vi "Bundle Script_In Place Insert.vi"(6 "Action Choice In":enum32{"Choice 1", "Choice 2"}(radio), 8 "error in":errorcluster, 10 "Selected Items Tags":string[](array[string]), 11 "Affected Items":T1) -> (0 "error out":errorcluster)   [LabVIEW 2023]
uses:
  top/BundleMagic.ctl
panel:
  # "Choice 1 is before, Choice 2 is after"
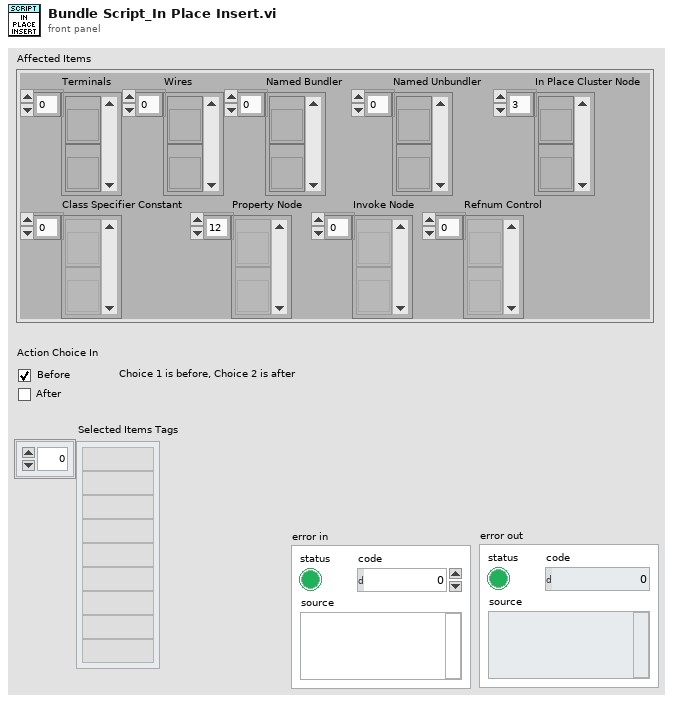
[diagram p1: front panel]
types:
  T1 = typedef "BundleMagic.ctl" = cluster{"Terminals":refnum<vi>[], "Wires":refnum<vi>[], "Named Bundler":refnum<vi>[], "Named Unbundler":refnum<vi>[], "In Place Cluster Node":refnum<vi>[], "Class Specifier Constant":refnum<vi>[], "Property Node":refnum<vi>[], "Invoke Node":refnum<vi>[], "Refnum Control":refnum<vi>[]}
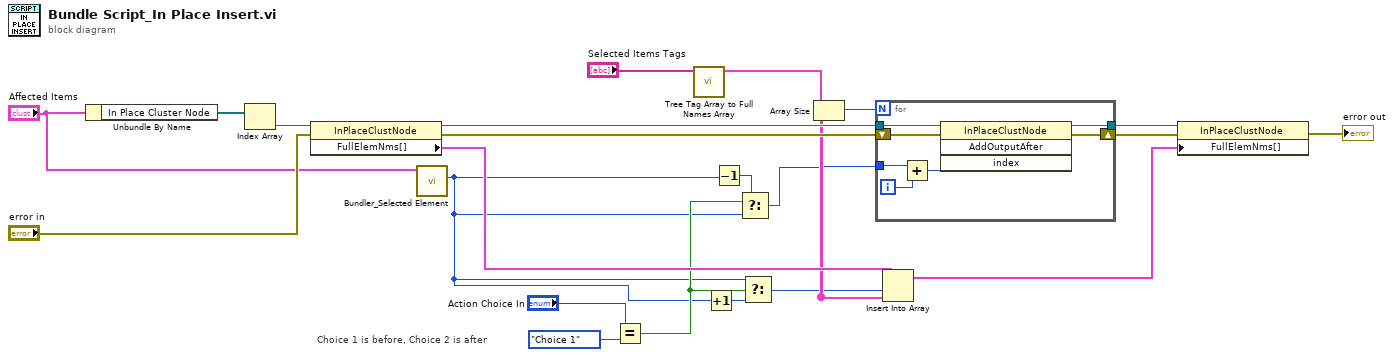
[diagram p0: block diagram]
diagram:
  # "Choice 1 is before, Choice 2 is after"
  n1 = Unbundle By Name("Affected Items") -> ("In Place Cluster Node"=w22:refnum<vi>[])
  n2 = Index Array(array=w22) -> (element=w19:refnum<vi>)  [unwired: 1 in]
  n3 = property class="InPlaceClustNode"(reference=w19, error in="error in") -> (reference out=w20:refnum<vi>, error out=w16:errorcluster, "FullElemNms[]"=w17:cluster{string[]}[])
  n4 = call "Bundler_Selected Element.vi"("Affected Items"="Affected Items") -> ("index of element"=w1:i32)  [unwired: 5 in, 5 out]
  n5 = Equal?(x="Action Choice In", y=enum32{"Choice 1", "Choice 2"}."Choice 1" ("Action Choice In")) -> (x = y?=w3:bool)
  n6 = call "Tree Tag Array to Full Names Array.vi"("Selected Items Tags"="Selected Items Tags") -> ("Tree Item Values (nested form)"=w13:cluster{"Array":string[]}[])  [unwired: 6 in, 4 out]
  n7 = Increment(x=w1) -> (x+1=w4:i32)
  n8 = Decrement(x=w1) -> (x-1=w7:i32)
  n9 = Select(t=w7, s=w3, f=w1) -> (s? t:f=w6:i32)
  n10 = Select(t=w1, s=w3, f=w4) -> (s? t:f=w5:i32)
  n11 = Array Size(array=w13) -> (size(s)=w10:i32)
  n12 = for {
    N: w10 -> [_]
    shift-right: [w27] -> w11
    shift-left: w16 -> [w28]
    tunnel: w20 -> [w26]
    tunnel: [w29] -> w12
    tunnel: w6 -> [w25]
    i -> [w24]
    n13 = Add(x=w25, y=w24) -> (x+y=w23:i32)
    n14 = invoke class="InPlaceClustNode" method="AddOutputAfter"(reference=w26, error in=w28, "index"=w23) -> (reference out=w29:refnum<vi>, error out=w27:errorcluster)  [unwired: 1 in, 2 out]
  }
  n15 = Insert Into Array(array=w17, index=w5, new element=w13) -> (w9:cluster{string[]}[])
  n16 = property class="InPlaceClustNode"(reference=w12, error in=w11, "FullElemNms[]"=w9) -> (error out=→"error out":errorcluster)  [unwired: 1 out]
